vi "V1 from String test.vi"() -> ()   [LabVIEW 2015, in "PID Module 2 tests.lvlib"]
uses:
  PID Module 2 tests.lvlib
  module/configuration/Line.ctl
  <vilib>/NI/Tag Bus Module Framework/channel/TBM channel.lvclass
  module/configuration/PID Module 2 configuration.lvclass
  module/configuration/PID Module 2 configuration.lvclass/PID Module 2 configuration.ctl
  <vilib>/NI/Tag Bus/tag/default value polymorphs/read default value Double.vi
  <vilib>/NI/Tag Bus/tag/tag descriptor.lvclass
  <vilib>/NI/Configuration Framework/serializable configuration/NISE_CEF_serializable configuration.lvclass
panel:
  out "PID ID":string
  out "Pass":bool
  out "Module Version":string
  out "error out":errorcluster
  out "D":dbl
  out "I":dbl
  out "P":dbl
  out "Low":dbl
  out "High":dbl
  out "Lines":T1[](array[typedef])
  in  "version":string="1.0.0.0"
  in  "data":string="<tbm_moduleversion>1.0.0</tbm_moduleversion>\r\n<tbm_moduledata><tbm_rootversion>1.0.0</tbm_rootversion>\r\n<tbm_rootdata>\r\n<instanceID>FF237443-909D-4B80-9254-0DF4E857D19F</instanceID>\r\n<kvpairs>\r\n<SCFG_AliasName>PID Module configuration</SCFG_AliasName>\r\n</kvpairs>\r\n</tbm_rootdata></tbm_moduledata>\r\n<my_pidloops><Test Loop><Test Loop_Setpoint>tag1</Test Loop_Setpoint>\r\n<Test Loop_ProcessVariable>tag2</Test Loop_ProcessVariable>\r\n<Test Loop_Output>tag3</Test Loop_Output>\r\n<Test Loop_Proportional>100.000000</Test Loop_Proportional>\r\n<Test Loop_Integral>200.000000</Test Loop_Integral>\r\n<Test Loop_Derivative>400.000000</Test Loop_Derivative>\r\n<Test Loop_RangeHigh>100.000000</Test Loop_RangeHigh>\r\n<Test Loop_RangeLow>-11.000000</Test Loop_RangeLow></Test Loop>\r\n</my_pidloops>"
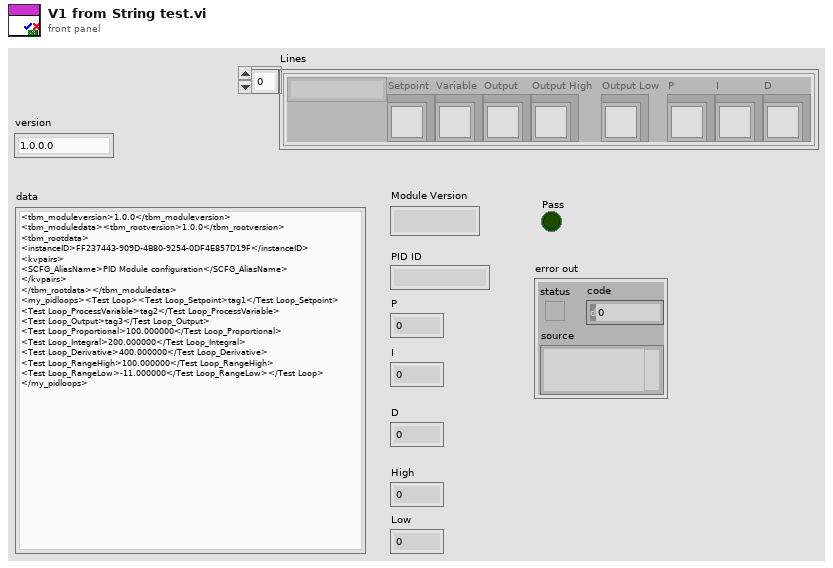
[diagram p1: front panel]
types:
  T1 = typedef "PID Module 2 configuration.lvclass/Line.ctl" = cluster{"PID ID":string, "Setpoint":refnum<class "TBM channel.lvclass">, "Variable":refnum<class "TBM channel.lvclass">, "Output":refnum<class "TBM channel.lvclass">, "Output High":refnum<class "TBM channel.lvclass">, "Output Low":refnum<class "TBM channel.lvclass">, "P":refnum<class "TBM channel.lvclass">, "I":refnum<class "TBM channel.lvclass">, "D":refnum<class "TBM channel.lvclass">}
  T2 = typedef "PID Loop.lvclass/PID Range.ctl" = cluster{"output high":dbl, "output low":dbl}
  T3 = typedef "PID Loop.lvclass/PID Gains.ctl" = cluster{"proportional gain (Kc)":dbl, "integral time (Ti, min)":dbl, "derivative time (Td, min)":dbl}
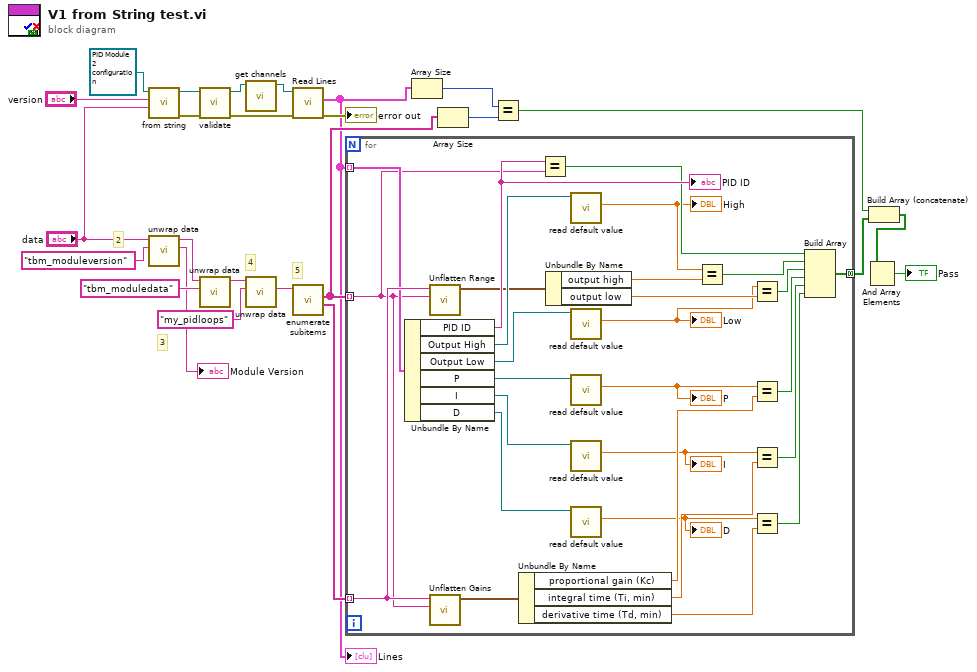
[diagram p0: block diagram]
diagram:
  # "5"
  # "4"
  # "3"
  # "2"
  n1 = call-dynamic "from string.vi"("data"="data", "version"="version", "PID Module 2 configuration in"=refnum<class "PID Module 2 configuration.lvclass"> refnum ("tag bus configurable plugin module configuration")) -> ("error out"=w20:errorcluster, "PID Module 2 configuration out"=w23:refnum<class "PID Module 2 configuration.lvclass">)  [unwired: 7 in]
  n2 = call <vilib>:"unwrap data.vi"("identifier"="tbm_moduleversion" ("additional identifier"), "data to unwrap"="data") -> ("unwrapped data"=→"Module Version":string, "remaining string"=w17:string)  [unwired: 8 in]
  n3 = call-dynamic "validate.vi"("error in"=w20, "PID Module 2 configuration in"=w23) -> ("error out"=w19:errorcluster, "PID Module 2 configuration out"=w22:refnum<class "PID Module 2 configuration.lvclass">)  [unwired: 8 in]
  n4 = call <vilib>:"unwrap data.vi"("identifier"="tbm_moduledata" ("additional identifier"), "data to unwrap"=w17) -> ("remaining string"=w14:string)  [unwired: 8 in, 1 out]
  n5 = call-dynamic "get channels.vi"("PID Module 2 configuration in"=w22) -> ("PID Module 2 configuration out"=w21:refnum<class "PID Module 2 configuration.lvclass">)  [unwired: 9 in, 1 out]
  n6 = call <vilib>:"unwrap data.vi"("identifier"="my_pidloops" ("additional identifier"), "data to unwrap"=w14) -> ("unwrapped data"=w12:string)  [unwired: 8 in, 1 out]
  n7 = call "Read Lines.vi"("error in (no error)"=w19, "PID Module 2 configuration in"=w21) -> ("error out"=→"error out":errorcluster, "Lines"=w4:T1[])  [unwired: 7 in, 1 out]
  "Lines" <- w4
  n8 = call <vilib>:"enumerate subitems.vi"("data to enumerate"=w12) -> ("associated data"=w11:string[], "discovered subitems"=w5:string[])  [unwired: 8 in, 1 out]
  n9 = for {
    tunnel: w5 -> [w45] mode=indexing
    tunnel: w11 -> [w53] mode=indexing
    tunnel: w4 -> [w47] mode=indexing
    tunnel: [w26] -> w7 mode=concatenating
    n10 = Unbundle By Name(w47) -> ("PID ID"=w46:string, "Output High"=w48:refnum<class "TBM channel.lvclass">, "Output Low"=w49:refnum<class "TBM channel.lvclass">, "P"=w50:refnum<class "TBM channel.lvclass">, "I"=w51:refnum<class "TBM channel.lvclass">, "D"=w52:refnum<class "TBM channel.lvclass">)
    "PID ID" <- w46
    n11 = call "Unflatten Range.vi"("Identifier"=w45, "Data to Unwrap"=w53) -> ("output range"=w33:T2)  [unwired: 9 in]
    n12 = call "Unflatten Gains.vi"("Identifier"=w45, "Data to Unwrap"=w53) -> ("PID gains"=w44:T3)  [unwired: 9 in]
    n13 = Unbundle By Name(w44) -> ("proportional gain (Kc)"=w43:dbl, "integral time (Ti, min)"=w41:dbl, "derivative time (Td, min)"=w39:dbl)
    n14 = Equal?(x=w46, y=w45) -> (x = y?=w34:bool)
    n15 = Unbundle By Name(w33) -> ("output high"=w32:dbl, "output low"=w30:dbl)
    n16 = call-poly <vilib>:"read default value.vi"("system tag in"=w48) -> ("default value"=w31:dbl)  [unwired: 7 in, 3 out]
    "High" <- w31
    n17 = call-poly <vilib>:"read default value.vi"("system tag in"=w49) -> ("default value"=w29:dbl)  [unwired: 7 in, 3 out]
    "Low" <- w29
    n18 = call-poly <vilib>:"read default value.vi"("system tag in"=w50) -> ("default value"=w42:dbl)  [unwired: 7 in, 3 out]
    "P" <- w42
    n19 = call-poly <vilib>:"read default value.vi"("system tag in"=w51) -> ("default value"=w40:dbl)  [unwired: 7 in, 3 out]
    "I" <- w40
    n20 = call-poly <vilib>:"read default value.vi"("system tag in"=w52) -> ("default value"=w38:dbl)  [unwired: 7 in, 3 out]
    "D" <- w38
    n21 = Equal?(x=w31, y=w32) -> (x = y?=w28:bool)
    n22 = Equal?(x=w29, y=w30) -> (x = y?=w27:bool)
    n23 = Equal?(x=w42, y=w43) -> (x = y?=w37:bool)
    n24 = Equal?(x=w40, y=w41) -> (x = y?=w36:bool)
    n25 = Equal?(x=w38, y=w39) -> (x = y?=w35:bool)
    n26 = Build Array(w34, w28, w27, w37, w36, w35) -> (w26:bool[])
  }
  n27 = Array Size(array=w4) -> (size(s)=w2:i32)
  n28 = Array Size(array=w5) -> (size(s)=w3:i32)
  n29 = Equal?(x=w2, y=w3) -> (x = y?=w1:bool)
  n30 = Build Array (concatenate)(w1, w7) -> (w6:bool[])
  n31 = And Array Elements(Boolean array=w6) -> (logical AND=→"Pass":bool)
